vi "getStatefromMemento.vi"(8 "error in (no error)":errorcluster, 10 "Memento In":refnum<class "Memento.lvclass">, 11 "Originator in":refnum<class "Originator.lvclass">) -> (0 "error out":errorcluster, 2 "State":string, 3 "Originator out":refnum<class "Originator.lvclass">)   [LabVIEW 2016, in "Originator.lvclass"]
uses:
  Originator.lvclass
  Memento Class/Memento.lvclass
  Memento Class/Memento.lvclass/Memento.ctl
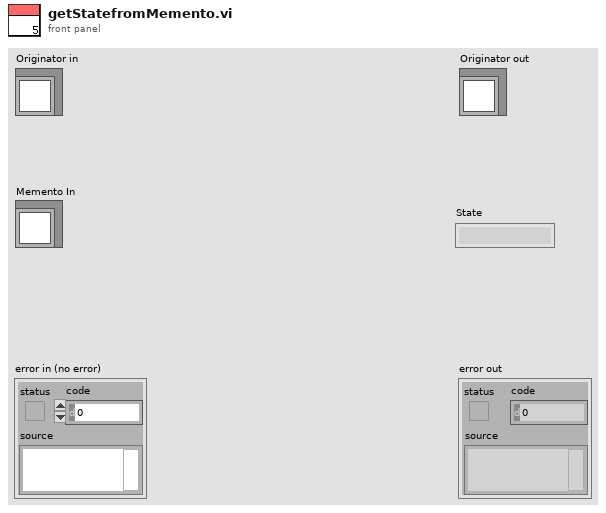
[diagram p1: front panel]
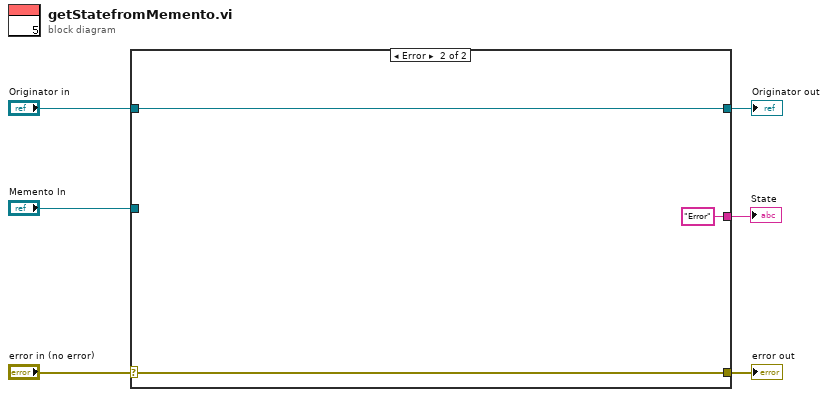
[diagram p0: block diagram]
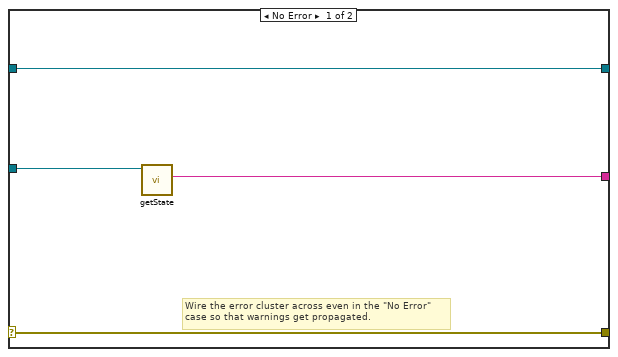
[diagram p2: hidden frame]
diagram:
  n1 = case shown="Error" "error in (no error)" {
    selector: "error in (no error)" -> [w9 w13]
    tunnel: [w9 w13] -> w5
    tunnel: [w10 w12] -> w3
    tunnel: "Originator in" -> [w10 w12]
    tunnel: "Memento In" -> [w8 _]
    tunnel: [w7 "Error" ("State")] -> w1
    frame No Error {
      # "Wire the error cluster across even in the \"No Error\"\ncase so that warnings get propagated."
      n2 = call "getState.vi"("Memento in"=w8) -> ("State"=w7:string)  [unwired: 8 in, 2 out]
    }
    frame Error {
    }
  }
  "error out" <- w5
  "Originator out" <- w3
  "State" <- w1
